vi "Get Target IP Address.vi"(8 "error in":errorcluster, 11 "Device Item Ref in":T1 format="%.0x") -> (0 "error out":errorcluster, 2 "IP Address":string, 3 "Item Ref out":T1 format="%.0x")   [LabVIEW 2019, in "TimingDRV System Explorer.lvlib"]
uses:
  TimingDRV System Explorer.lvlib
  <vilib>/NI VeriStand/Custom Device API/Custom Device Item Ref.ctl
  NationalInstruments.VeriStand.SystemDefinitionAPI
  NationalInstruments.VeriStand.SystemStorage
  <vilib>/NI VeriStand/Custom Device Tools/Custom Device Utility Library/Custom Device Utility Library.lvlib
  <vilib>/NI VeriStand/Custom Device API/Custom Device API.lvlib
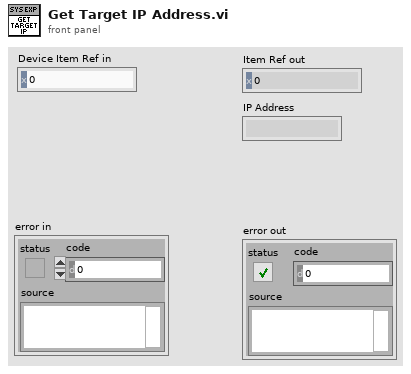
[diagram p1: front panel]
types:
  T1 = typedef "Custom Device API.lvlib/Custom Device Item Ref.ctl" = u64
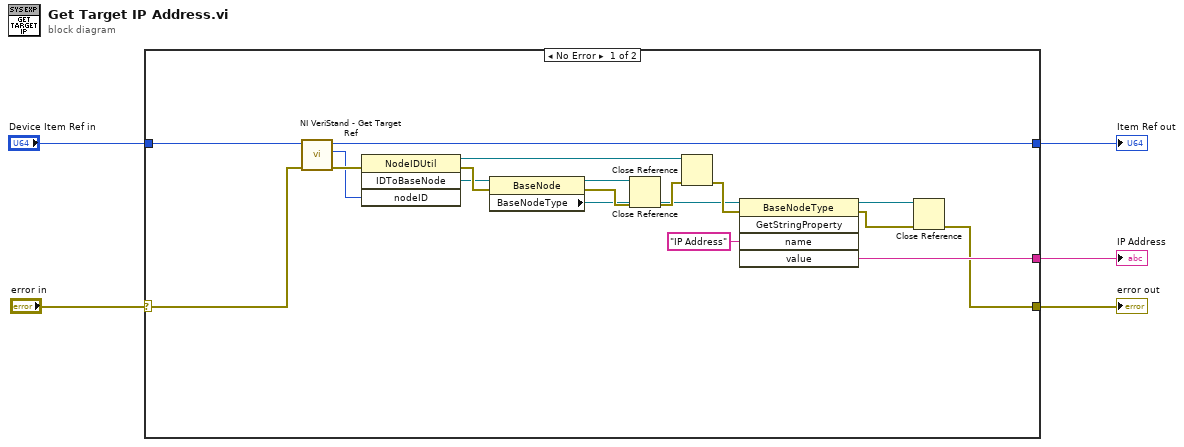
[diagram p0: block diagram]
diagram:
  n1 = case shown="No Error" "error in" {
    selector: "error in" -> [w6 w25]
    tunnel: [w23 w24] -> w5
    tunnel: "Device Item Ref in" -> [w22 w24]
    tunnel: [w21 _] -> w3
    tunnel: [w7 w25] -> w2
    frame No Error {
      n2 = call <vilib>:"NI VeriStand - Get Target Ref.vi"("error in"=w6, "Item Ref in"=w22) -> ("error out"=w13:errorcluster, "Target Ref"=w10:T1, "Item Ref out"=w23:T1)  [unwired: 6 in, 1 out]
      n3 = invoke class="NodeIDUtil" method="IDToBaseNode"(error in=w13, "nodeID"=w10) -> (reference out=w16:refnum<k24>, error out=w15:errorcluster, "IDToBaseNode"=w14:refnum<k24>)  [unwired: 2 in, 1 out]
      n4 = property class="BaseNode"(reference=w14, error in=w15) -> (reference out=w18:refnum<k24>, error out=w17:errorcluster, "BaseNodeType"=w11:refnum<k24>)
      n5 = Close Reference(reference=w18, error in (no error)=w17) -> (error out=w19:errorcluster)
      n6 = Close Reference(reference=w16, error in (no error)=w19) -> (error out=w12:errorcluster)
      n7 = invoke class="BaseNodeType" method="GetStringProperty"(reference=w11, error in=w12, "name"="IP Address") -> (reference out=w8:refnum<k24>, error out=w9:errorcluster, "value"=w21:string)  [unwired: 2 in, 2 out]
      n8 = Close Reference(reference=w8, error in (no error)=w9) -> (error out=w7:errorcluster)
    }
    frame Error {
    }
  }
  "Item Ref out" <- w5
  "IP Address" <- w3
  "error out" <- w2
